vi "Host Interface.vi"(5 "High Address":u32=3225485311 format="%08x", 7 "Base Address":u32=3225419776 format="%08x") -> (0 "Write error?":bool, 1 "Read Error?":bool, 3 "CS?":bool)   [LabVIEW 2011]
uses:
  <vilib>/Platform/TimedLoop/XDataNode/timing_clust.ctl
  <vilib>/Platform/TimedLoop/XDataNode/nitl_modes.ctl
  <vilib>/Platform/TimedLoop/XDataNode/wakeup.ctl
  <vilib>/rvi/eio/common/nirviEmuTemplateMethod_errors.vi
  <vilib>/Platform/TimedLoop/XDataNode/XDataNode.xnode
  <vilib>/eio/EIONode/EIONode.xnode
  <vilib>/Platform/TimedLoop/XDataNode/XDNodeRunTimeDep.lvlib
panel:
  out "Read offset":u32 format="%08x"
  out "Read data":u32 format="%08x"
  out "Write offset":u32 format="%08x"
  out "Write data":u32 format="%08x"
  out "Byte enable?":bool[](array[boolean])
  out "Address":u32 format="%08x"
  out "Read?":bool
  out "Reset?":bool
  # "Host Interface"
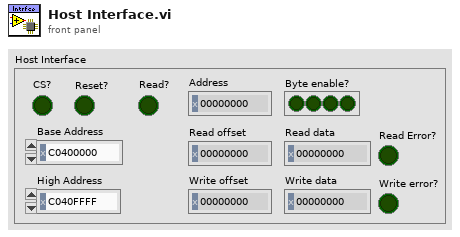
[diagram p1: front panel]
types:
  T1 = typedef "XDNodeRunTimeDep.lvlib/timing_clust.ctl" = cluster{"Expected End [f-1]":u64, "Actual End [f-1]":u64, "Finished Late? [f-1]":bool, "Expected End [i-1]":u64, "Actual End [i-1]":u64, "Finished Late? [i-1]":bool, "Expected Start [i]":u64, "Actual Start [i]":u64, "Expected Start [f]":u64, "Actual Start [f]":u64, "Source Name":string, "Structure Name":string, "Period":i64, "Deadline":i64, "Offset":i64, "Start":i64, "Priority":i32, "Timeout":i32, "Mode":T2, "Wakeup Reason":T3, "Error":errorcluster, "Source Type":string, "Secondary Source Type":string, "Global End Time":u64, "Global Start Time":u64, "Frame Duration":u64, "Iteration Duration":u64, "Assigned CPU":i32, "I/O Scan Engine Mode":u32}
  T2 = typedef "XDNodeRunTimeDep.lvlib/nitl_modes.ctl" = enum32{"No Change", "Process missed periods, maintain original phase", "Discard missed periods, maintain original phase", "Process missed periods, ignore original phase", "Discard missed periods, ignore original phase"}
  T3 = typedef "XDNodeRunTimeDep.lvlib/wakeup.ctl" = enum32{"Normal", "Aborted", "Asynchronous wakeup", "Timing source error", "Timed loop error", "Timeout"}
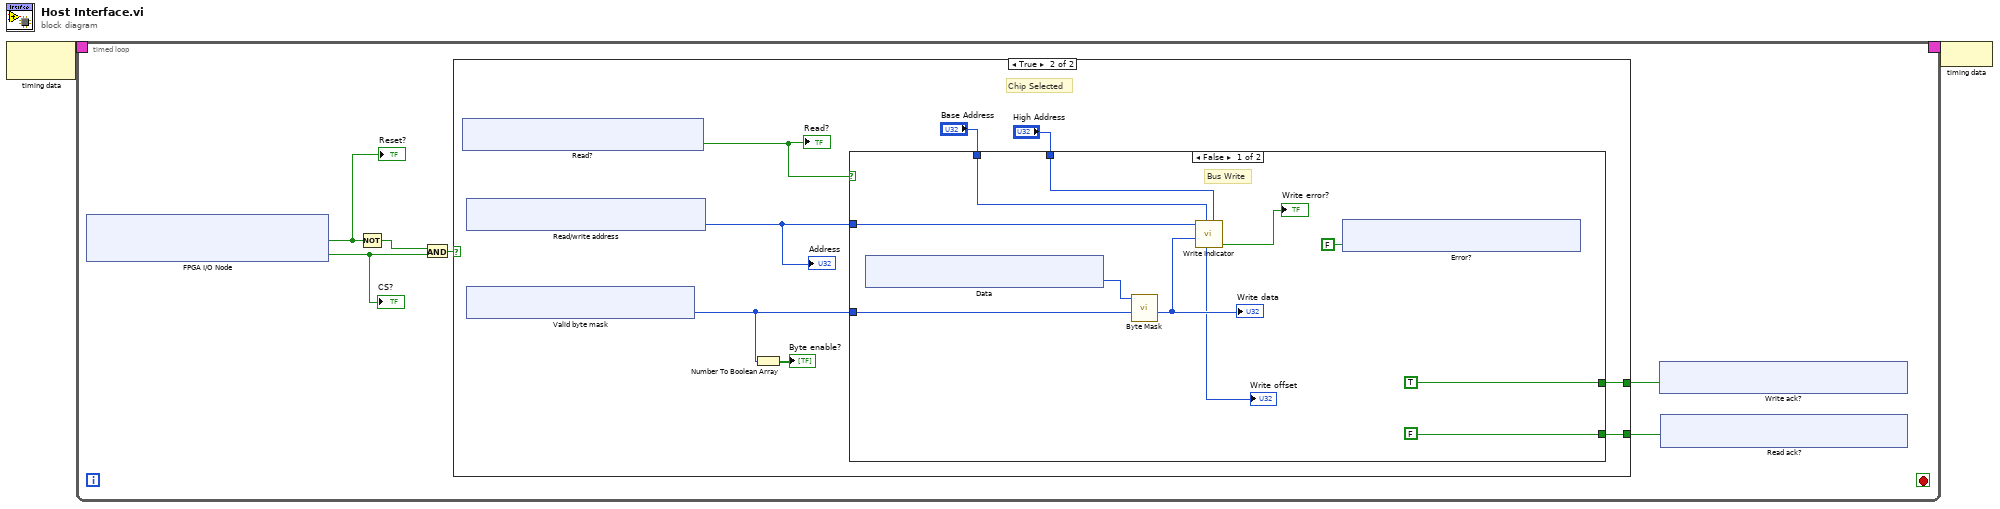
[diagram p0: block diagram]
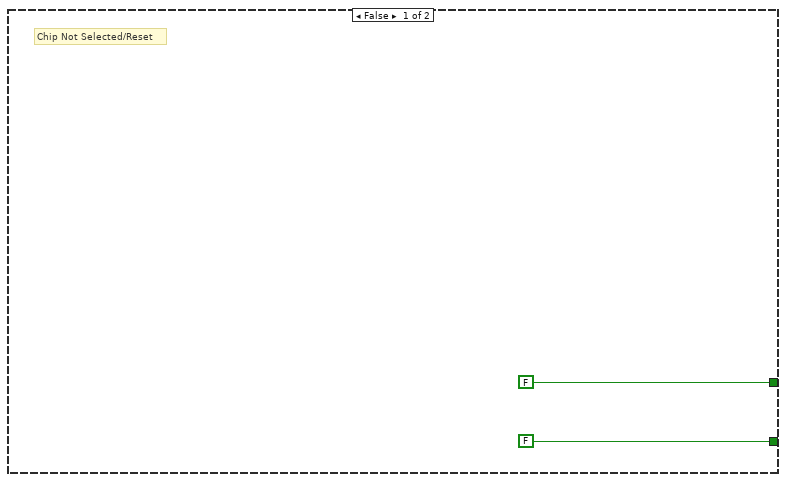
[diagram p2: hidden frame]
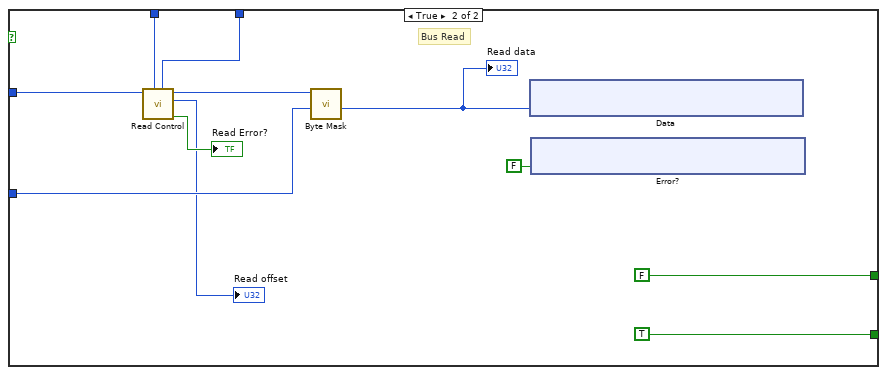
[diagram p3: hidden frame]
diagram:
  n1 = node-c288() -> (w2:T1)  [unwired: 1 in]
  n2 = timed-loop {
    timing: w2 -> [_]
    timing-out: [_] -> w1
    stop <- _ stop-if-true
    n3 = xnode "FPGA I/O Node"() -> ("microblaze\\ipic_test_0_ipif_Bus2IP_Reset_pin"=w7:bool, "microblaze\\ipic_test_0_ipif_Bus2IP_CS_pin"=w5:bool)  [unwired: 2 in, 2 out]
    "CS?" <- w5
    "Reset?" <- w7
    n4 = Not(x=w7) -> (.not. x?=w6:bool)
    n5 = And(x=w6, y=w5) -> (x .and. y?=w8:bool)
    n6 = case shown="True" w8 {
      tunnel: [FALSE ("myprocessor\\ipic_test_0_ipif_IP2Bus_WrAck_pin") w12] -> w4
      tunnel: [FALSE ("myprocessor\\ipic_test_0_ipif_IP2Bus_RdAck_pin") w11] -> w3
      frame False {
        # "Chip Not Selected/Reset"
      }
      frame True {
        # "Chip Selected"
        n7 = xnode "Read?"() -> ("microblaze\\ipic_test_0_ipif_Bus2IP_RNW_pin"=w18:bool)  [unwired: 1 in, 1 out]
        "Read?" <- w18
        n8 = xnode "Read/write address"() -> ("microblaze\\ipic_test_0_ipif_Bus2IP_Addr_pin"=w17:i32)  [unwired: 1 in, 1 out]
        "Address" <- w17
        n9 = xnode "Valid byte mask"() -> ("microblaze\\ipic_test_0_ipif_Bus2IP_BE_pin"=w15:i8)  [unwired: 1 in, 1 out]
        n10 = Number To Boolean Array(number=w15) -> (Boolean array=→"Byte enable?":bool[])
        n11 = case shown="False" w18 {
          tunnel: w17 -> [w29 w40]
          tunnel: w15 -> [w27 w38]
          tunnel: "Base Address" -> [w25 w36]
          tunnel: "High Address" -> [w24 w37]
          tunnel: [TRUE ("myprocessor\\ipic_test_0_ipif_IP2Bus_WrAck_pin") FALSE ("myprocessor\\ipic_test_0_ipif_IP2Bus_WrAck_pin")] -> w12
          tunnel: [FALSE ("myprocessor\\ipic_test_0_ipif_IP2Bus_RdAck_pin") TRUE ("myprocessor\\ipic_test_0_ipif_IP2Bus_RdAck_pin")] -> w11
          frame False {
            # "Bus Write"
            n12 = xnode "Data"() -> ("microblaze\\ipic_test_0_ipif_Bus2IP_Data_pin"=w28:i32)  [unwired: 1 in, 1 out]
            n13 = call "Byte Mask.vi"("Byte Mask"=w27, "Data"=w28) -> ("Masked Data"=w20:u32)  [unwired: 9 in]
            "Write data" <- w20
            n14 = call "Write Indicator.vi"("High Address"=w24, "Base Address"=w25, "Data"=w20, "Address"=w29) -> ("Error?"=→"Write error?":bool, "Offset"=→"Write offset":u32)  [unwired: 6 in]
            n15 = xnode "Error?"("microblaze\\ipic_test_0_ipif_IP2Bus_Error_pin"=FALSE ("myprocessor\\ipic_test_0_ipif_IP2Bus_Error_pin")) -> ()  [unwired: 1 in, 1 out]
          }
          frame True {
            # "Bus Read"
            n16 = call "Read Control.vi"("High Address"=w37, "Base Address"=w36, "Address"=w40) -> ("Error?"=→"Read Error?":bool, "Offset"=→"Read offset":u32, "Data"=w39:i32)  [unwired: 6 in]
            n17 = call "Byte Mask.vi"("Byte Mask"=w38, "Data"=w39) -> ("Masked Data"=w31:u32)  [unwired: 9 in]
            "Read data" <- w31
            n18 = xnode "Data"("microblaze\\ipic_test_0_ipif_IP2Bus_Data_pin"=w31) -> ()  [unwired: 1 in, 1 out]
            n19 = xnode "Error?"("microblaze\\ipic_test_0_ipif_IP2Bus_Error_pin"=FALSE ("myprocessor\\ipic_test_0_ipif_IP2Bus_Error_pin")) -> ()  [unwired: 1 in, 1 out]
          }
        }
      }
    }
    n20 = xnode "Write ack?"("microblaze\\ipic_test_0_ipif_IP2Bus_WrAck_pin"=w4) -> ()  [unwired: 1 in, 1 out]
    n21 = xnode "Read ack?"("microblaze\\ipic_test_0_ipif_IP2Bus_RdAck_pin"=w3) -> ()  [unwired: 1 in, 1 out]
  }
  n22 = node-c288(w1) -> ()
